vi "FlpLib IIRDirectFormIITrans2ndOrder 0.vi"(0 "xn":sgl, 1 "ak":sgl[](array[numeric])=[0.0, 0.0], 2 "bk":sgl[](array[numeric])=[0.0, 0.0, 0.0], 11 "stateIn":sgl[](array[numeric])=[0.0, 0.0]) -> (4 "yn":sgl, 15 "stateOut":sgl[](array[numeric]))   [LabVIEW 2017]
uses:
  <userlib>/_NI FLP Library/FPGA/outsideSCTL/FlpLib Multiply Shared Instance 0.vi
  <userlib>/_NI FLP Library/FPGA/outsideSCTL/FlpLib Add Shared Instance 0.vi
  <userlib>/_NI FLP Library/FPGA/outsideSCTL/FlpLib Subtract Shared Instance 0.vi
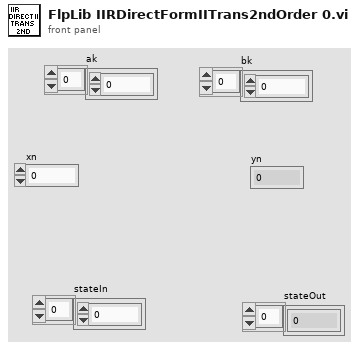
[diagram p1: front panel]
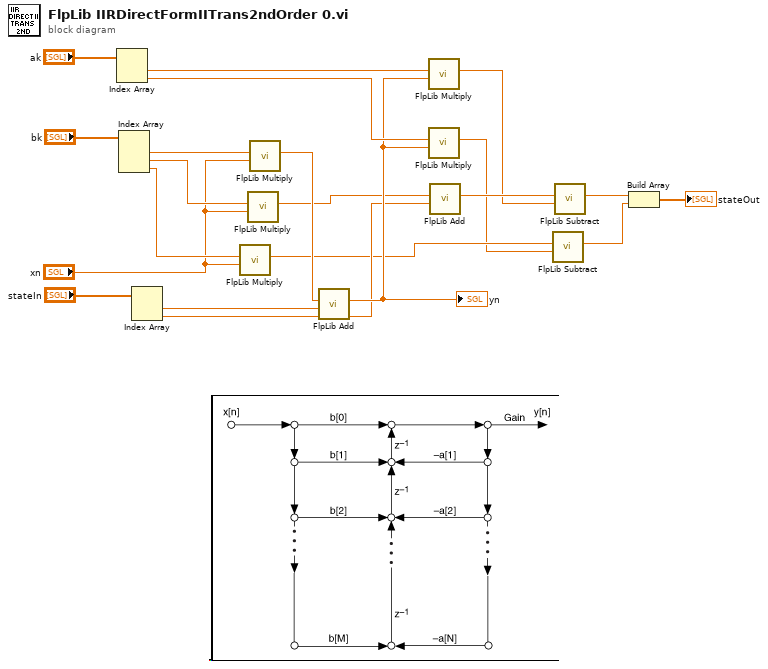
[diagram p0: block diagram]
diagram:
  n1 = Index Array(array="ak") -> (element #1=w12:sgl, element #2=w11:sgl)  [unwired: 2 in]
  n2 = Index Array(array="bk") -> (element #1=w18:sgl, element #2=w17:sgl, element #3=w16:sgl)  [unwired: 3 in]
  n3 = Index Array(array="stateIn") -> (element #1=w14:sgl, element #2=w8:sgl)  [unwired: 2 in]
  n4 = call-poly <userlib>:"FlpLib Multiply.vi"("y"="xn", "x"=w16) -> ("x*y"=w4:sgl)  [unwired: 5 in]
  n5 = call-poly <userlib>:"FlpLib Multiply.vi"("y"="xn", "x"=w17) -> ("x*y"=w9:sgl)  [unwired: 5 in]
  n6 = call-poly <userlib>:"FlpLib Multiply.vi"("y"="xn", "x"=w18) -> ("x*y"=w13:sgl)  [unwired: 5 in]
  n7 = call-poly <userlib>:"FlpLib Add.vi"("y"=w14, "x"=w13) -> ("x+y"=w10:sgl)  [unwired: 5 in]
  "yn" <- w10
  n8 = call-poly <userlib>:"FlpLib Multiply.vi"("y"=w10, "x"=w12) -> ("x*y"=w6:sgl)  [unwired: 5 in]
  n9 = call-poly <userlib>:"FlpLib Multiply.vi"("y"=w10, "x"=w11) -> ("x*y"=w3:sgl)  [unwired: 5 in]
  n10 = call-poly <userlib>:"FlpLib Add.vi"("y"=w8, "x"=w9) -> ("x+y"=w7:sgl)  [unwired: 5 in]
  n11 = call-poly <userlib>:"FlpLib Subtract.vi"("y"=w3, "x"=w4) -> ("x-y"=w2:sgl)  [unwired: 5 in]
  n12 = call-poly <userlib>:"FlpLib Subtract.vi"("y"=w6, "x"=w7) -> ("x-y"=w5:sgl)  [unwired: 5 in]
  n13 = Build Array(w5, w2) -> (→"stateOut":sgl[])
